vi "Item_Init.vi"(11 "Object":T1) -> ()   [LabVIEW 2020, in "Project Provider.lvlib"]
uses:
  Project Provider.lvlib
  <resource>/Framework/Providers/API/ItemRef.ctl
  Framework/Mock/LMock Mock.lvclass
  <resource>/Framework/Providers/API/mxLvOverlayState.ctl
  <resource>/Framework/Providers/API/mxLvUpdateUI.ctl
panel:
  out "error out":errorcluster
  in  "error in":errorcluster
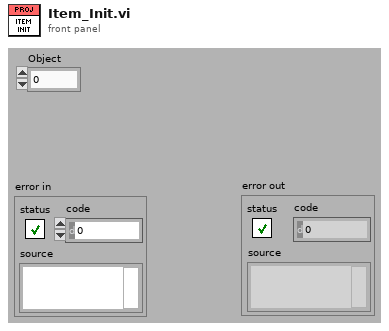
[diagram p1: front panel]
types:
  T1 = typedef "ItemRef.ctl" = u64
  T2 = typedef "mxLvOverlayState.ctl" = cluster{"Overlay Alias":string, "Active":bool}
  T3 = typedef "mxLvUpdateUI.ctl" = cluster{"Action":u32, "Optional param 1":string, "Optional param 2":i32, "Optional param 3":string}
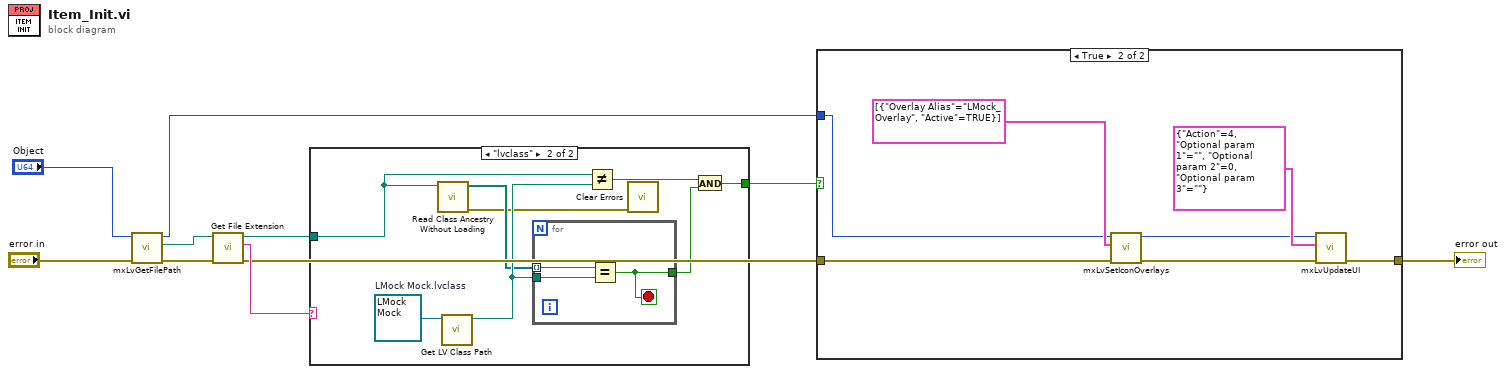
[diagram p0: block diagram]
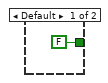
[diagram p3: hidden frame]
diagram:
  n1 = call <resource>:"mxLvGetFilePath.vi"("error in"="error in", "Item"="Object") -> ("error out"=w7:errorcluster, "File Path"=w6:path, "Item"=w2:T1)  [unwired: 7 in]
  n2 = call <vilib>:"Get File Extension.vi"("error in (no error)"=w7, "file"=w6) -> ("error out"=w3:errorcluster, "lowercase file extension"=w4:string, "dup file"=w5:path)  [unwired: 5 in, 2 out]
  n3 = case shown="\"lvclass\"" w4 {
    tunnel: w5 -> [_ w13]
    tunnel: [FALSE w12] -> w1
    frame Default {
    }
    frame "lvclass" {
      w19 = refnum<class "LMock Mock.lvclass"> refnum  # LMock Mock.lvclass
      n4 = call <vilib>:"Read Class Ancestry Without Loading.vi"("LabVIEW Class Path"=w13) -> ("error out"=w15:errorcluster, "Class Ancestry"=w17:path[])  [unwired: 9 in]
      n5 = call <vilib>:"Get LV Class Path.vi"("object"=w19) -> ("class path"=w18:path)  [unwired: 9 in, 1 out]
      n6 = for {
        tunnel: w17 -> [w22] mode=indexing
        tunnel: w18 -> [w21]
        tunnel: [w20] -> w16
        stop <- w20 stop-if-true
        n7 = Equal?(x=w22, y=w21) -> (x = y?=w20:bool)
      }
      n8 = Not Equal?(x=w13, y=w18) -> (x != y?=w14:bool)
      n9 = call <vilib>:"Clear Errors.vi"("error in (no error)"=w15) -> ()  [unwired: 5 in, 2 out]
      n10 = And(x=w14, y=w16) -> (x .and. y?=w12:bool)
    }
  }
  n11 = case shown="True" w1 {
    tunnel: w3 -> [w23 w28]
    tunnel: [w23 w26] -> w8
    tunnel: w2 -> [_ w25]
    frame False {
    }
    frame True {
      n12 = call <resource>:"mxLvSetIconOverlays.vi"("error in"=w28, "Overlay States"=T2[] [{"Overlay Alias"="LMock_Overlay", "Active"=TRUE}] ("Array"), "Item"=w25) -> ("error out"=w27:errorcluster, "Item"=w24:T1)  [unwired: 7 in]
      n13 = call <resource>:"mxLvUpdateUI.vi"("error in"=w27, "Update UI Settings"=T3 {"Action"=4, "Optional param 1"="", "Optional param 2"=0, "Optional param 3"=""}, "Item"=w24) -> ("error out"=w26:errorcluster)  [unwired: 7 in, 1 out]
    }
  }
  "error out" <- w8
